vi "HXG2_Analog-IN_PROCESS.vi"(8 "error in (no error)":errorcluster, 10 "Analog TC":dbl[][](array[numeric]) format="%0.2f", 11 "Analog In":dbl[][](array[numeric]) format="%0.2f") -> (0 "error out":errorcluster, 3 "ANALOG OUT":T1)   [LabVIEW 2012]
uses:
  Controls/HXG2_AnalogIn.ctl
  <vilib>/Analysis/Matrix/Numeric/Conversions/Array To Matrix - RA2.vi
  <vilib>/Analysis/baseanly.llb/A x Vector.vi
  <vilib>/Analysis/NI_AALBase.lvlib
  <vilib>/Analysis/Matrix/NI_Matrix.lvlib
panel:
  out "TC Samples":i32
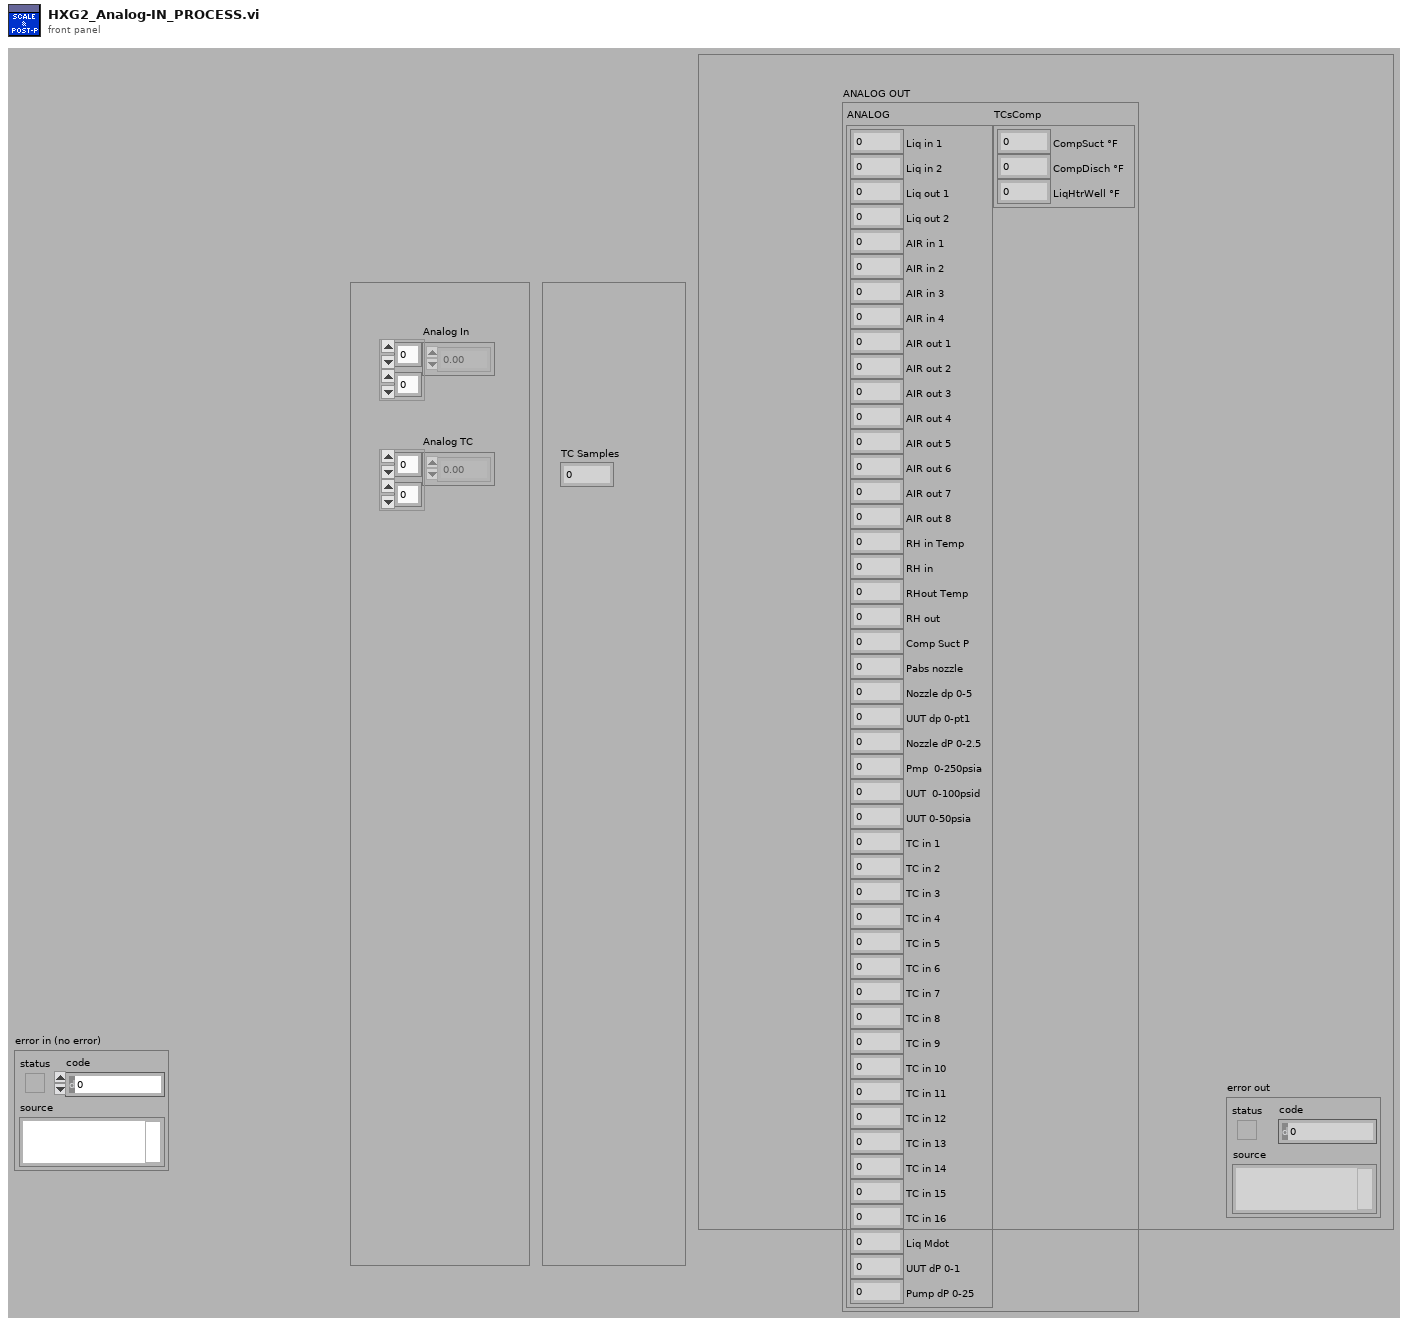
[diagram p1: front panel]
types:
  T1 = typedef "HXG2_AnalogIn.ctl" = cluster{"ANALOG":cluster{"Liq in 1":dbl, "Liq in 2":dbl, "Liq out 1":dbl, "Liq out 2":dbl, "AIR in 1":dbl, "AIR in 2":dbl, "AIR in 3":dbl, "AIR in 4":dbl, "AIR out 1":dbl, "AIR out 2":dbl, "AIR out 3":dbl, "AIR out 4":dbl, "AIR out 5":dbl, "AIR out 6":dbl, "AIR out 7":dbl, "AIR out 8":dbl, "RH in Temp":dbl, "RH in":dbl, "RHout Temp":dbl, "RH out":dbl, "Comp Suct P":dbl, "Pabs nozzle":dbl, "Nozzle dp 0-5":dbl, "UUT dp 0-pt1":dbl, "Nozzle dP 0-2.5":dbl, "Pmp  0-250psia":dbl, "UUT  0-100psid":dbl, "UUT 0-50psia":dbl, "TC in 1":dbl, "TC in 2":dbl, "TC in 3":dbl, "TC in 4":dbl, "TC in 5":dbl, "TC in 6":dbl, "TC in 7":dbl, "TC in 8":dbl, "TC in 9":dbl, "TC in 10":dbl, "TC in 11":dbl, "TC in 12":dbl, "TC in 13":dbl, "TC in 14":dbl, "TC in 15":dbl, "TC in 16":dbl, "Liq Mdot":dbl, "UUT dP 0-1":dbl, "Pump dP 0-25":dbl}, "TCsComp":cluster{"CompSuct °F  ":dbl, "CompDisch °F":dbl, "LiqHtrWell °F":dbl}}
  T2 = typedef "NI_Matrix.lvlib/RealMatrix.ctl" = dbl[][]
  T3 = cluster{"Analog TC[0]":dbl, "Analog TC[1]":dbl, "Analog TC[2]":dbl, "Analog TC[3]":dbl, "Analog TC[4]":dbl}
  T4 = cluster{"[0]":dbl, "[1]":dbl, "[2]":dbl, "[3]":dbl, "[4]":dbl, "[5]":dbl, "[6]":dbl, "[7]":dbl, "[8]":dbl, "[9]":dbl, "[10]":dbl, "[11]":dbl, "[12]":dbl, "[13]":dbl, "[14]":dbl, "[15]":dbl, "[16]":dbl, "[17]":dbl, "[18]":dbl, "[19]":dbl, "[20]":dbl, "[21]":dbl, "[22]":dbl, "[23]":dbl, "[24]":dbl, "[25]":dbl, "[26]":dbl, "[27]":dbl, "[28]":dbl, "[29]":dbl, "[30]":dbl, "[31]":dbl, "[32]":dbl, "[33]":dbl, "[34]":dbl, "[35]":dbl, "[36]":dbl, "[37]":dbl, "[38]":dbl, "[39]":dbl, "[40]":dbl, "[41]":dbl, "[42]":dbl, "[43]":dbl, "[44]":dbl, "[45]":dbl, "[46]":dbl}
  T5 = cluster{"Analog TC[0]":dbl, "Analog TC[1]":dbl, "Analog TC[2]":dbl}
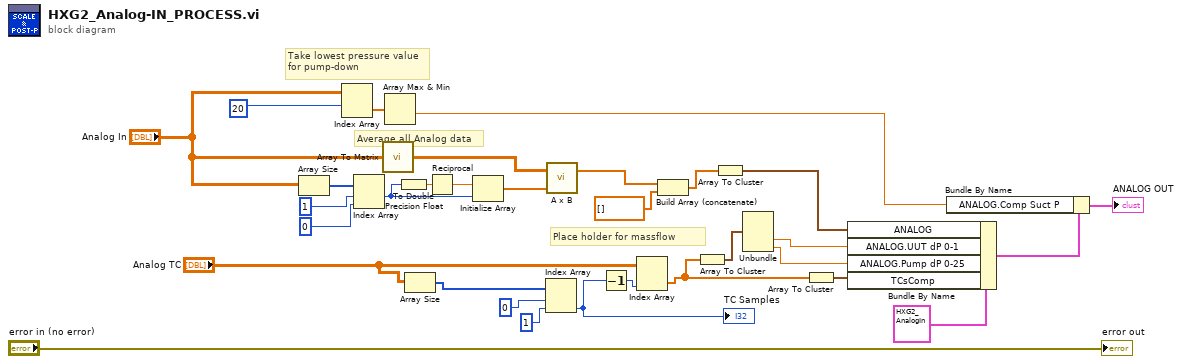
[diagram p0: block diagram]
diagram:
  # "Place holder for massflow"
  # "Take lowest pressure value\nfor pump-down"
  # "Average all Analog data"
  n1 = Array Size(array="Analog In") -> (size(s)=w20:i32[])
  n2 = Index Array(array="Analog In", index (row)=20) -> (element=w24:dbl[])  [unwired: 1 in]
  n3 = Index Array(array=w20, index #1=1 ("index"), index #2=0 ("index")) -> (element #1=w28:i32)  [unwired: 1 out]
  n4 = call-poly <vilib>:"Array To Matrix.vi"("Real 2D Array"="Analog In") -> ("Real Matrix"=w17:T2)
  n5 = Array Max & Min(array=w24) -> (min value=w31:dbl)  [unwired: 3 out]
  n6 = To Double Precision Float(number=w28) -> (double precision float=w18:dbl)
  n7 = Array Size(array="Analog TC") -> (size(s)=w15:i32[])
  n8 = Reciprocal(x=w18) -> (1/x=w19:dbl)
  n9 = Initialize Array(w19, w28) -> (w27:dbl[])
  n10 = Index Array(array=w15, index #1=0 ("index"), index #2=1 ("index")) -> (element #2=w7:i32)  [unwired: 1 out]
  "TC Samples" <- w7
  n11 = call-poly <vilib>:"A x B.vi"("Vector"=w27, "A"=w17) -> ("A x Vector"=w9:dbl[])  [unwired: 1 out]
  n12 = Decrement(x=w7) -> (x-1=w6:i32)
  n13 = Index Array(array="Analog TC", index (col)=w6) -> (element=w4:dbl[])  [unwired: 1 in]
  n14 = Build Array (concatenate)(w9, dbl[] [] ("array")) -> (w8:dbl[])
  n15 = Array To Cluster(array=w4) -> (cluster=w3:T3)
  n16 = Array To Cluster(array=w8) -> (cluster=w23:T4)
  n17 = Unbundle(w3) -> ("Analog TC[3]"=w2:dbl, "Analog TC[4]"=w1:dbl)  [unwired: 3 out]
  n18 = Array To Cluster(array=w4) -> (cluster=w5:T5)
  n19 = Bundle By Name(cluster=T1 {"ANALOG"={"Liq in 1"=0.0, "Liq in 2"=0.0, "Liq out 1"=0.0, "Liq out 2"=0.0, "AIR in 1"=0.0, "AIR in 2"=0.0, "AIR in 3"=0.0, "AIR in 4"=0.0, "AIR out 1"=0.0, "AIR out 2"=0.0, "AIR out 3"=0.0, "AIR out 4"=0.0, "AIR out 5"=0.0, "AIR out 6"=0.0, "AIR out 7"=0.0, "AIR out 8"=0.0, "RH in Temp"=0.0, "RH in"=0.0, "RHout Temp"=0.0, "RH out"=0.0, "Comp Suct P"=0.0, "Pabs nozzle"=0.0, "Nozzle dp 0-5"=0.0, "UUT dp 0-pt1"=0.0, "Nozzle dP 0-2.5"=0.0, "Pmp  0-250psia"=0.0, "UUT  0-100psid"=0.0, "UUT 0-50psia"=0.0, "TC in 1"=0.0, "TC in 2"=0.0, "TC in 3"=0.0, "TC in 4"=0.0, "TC in 5"=0.0, "TC in 6"=0.0, "TC in 7"=0.0, "TC in 8"=0.0, "TC in 9"=0.0, "TC in 10"=0.0, "TC in 11"=0.0, "TC in 12"=0.0, "TC in 13"=0.0, "TC in 14"=0.0, "TC in 15"=0.0, "TC in 16"=0.0, "Liq Mdot"=0.0, "UUT dP 0-1"=0.0, "Pump dP 0-25"=0.0}, "TCsComp"={"CompSuct °F  "=0.0, "CompDisch °F"=0.0, "LiqHtrWell °F"=0.0}} ("DATA In"), "ANALOG"=w23, "ANALOG.UUT dP 0-1"=w2, "ANALOG.Pump dP 0-25"=w1, "TCsComp"=w5) -> (w29:T1)
  n20 = Bundle By Name(cluster=w29, "ANALOG.Comp Suct P"=w31) -> (→"ANALOG OUT":T1)
  "error out" <- "error in (no error)"
